vi "Format CSV.vi"(8 "error in (no error)":errorcluster, 9 "delimiter":string=",", 10 "CSV File Input":path, 11 "Original CSV Format":enum16{"Format A", "Format B"}(ring)) -> (0 "error out":errorcluster, 1 "Parcel Length":i32[](array[numeric]), 2 "All Terminal Data":T1(array[cluster]))   [LabVIEW 2017] (continued)
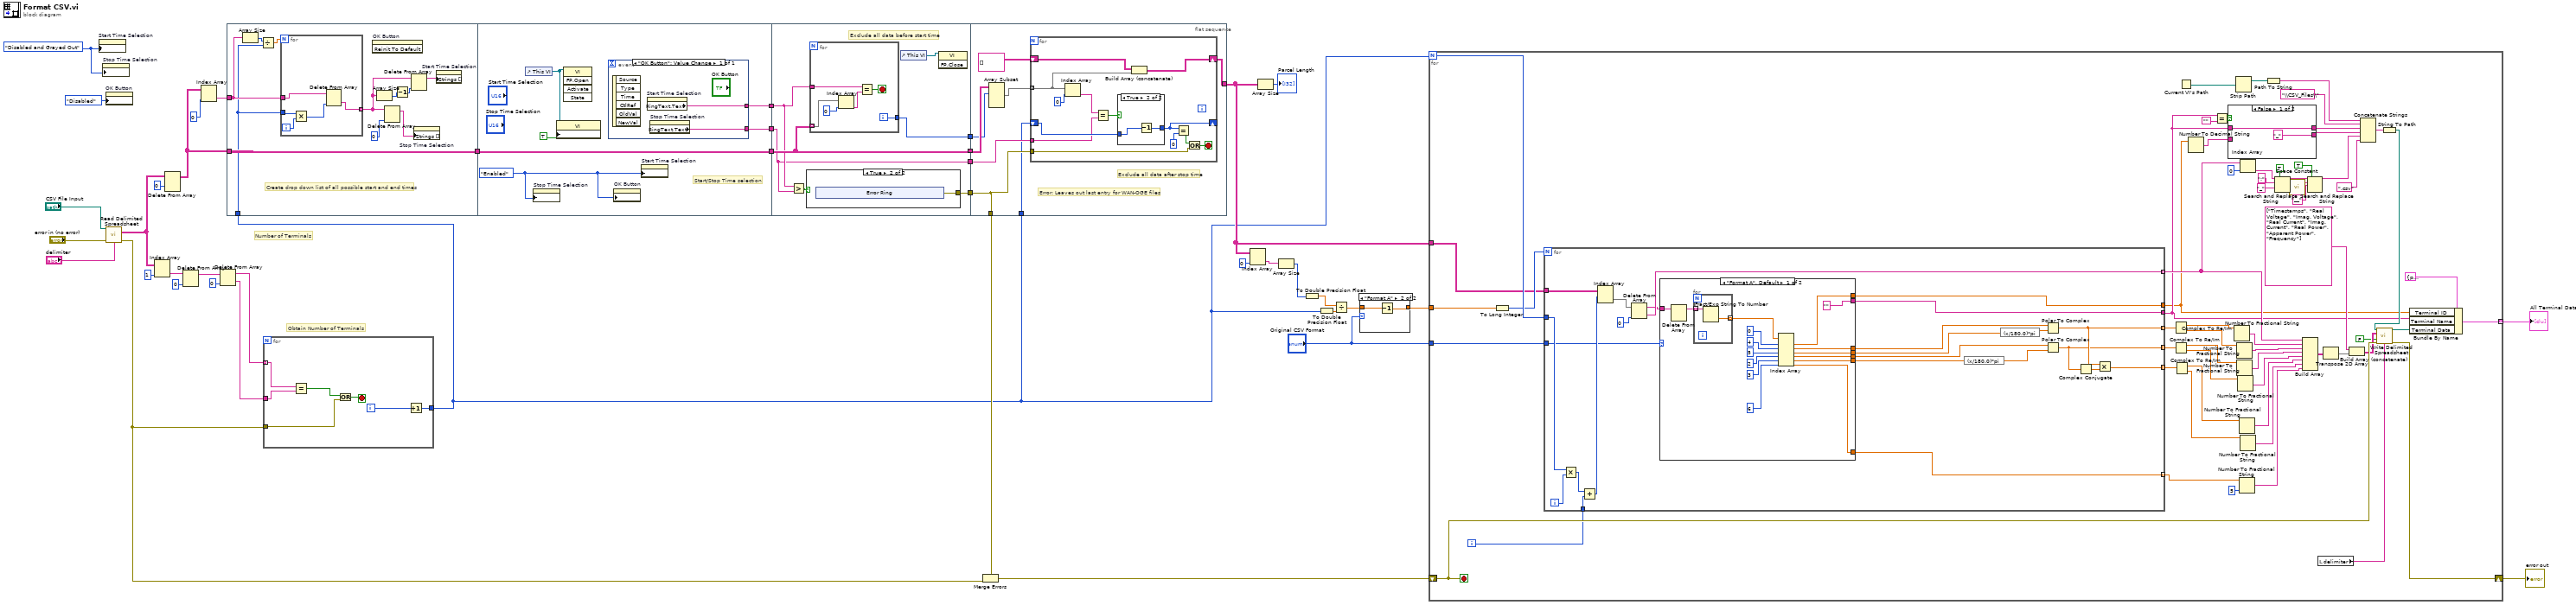
[diagram p0: block diagram]
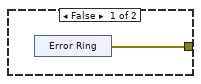
[diagram p3: hidden frame]
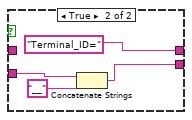
[diagram p5: hidden frame]
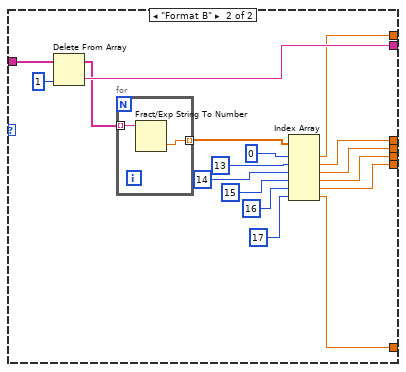
[diagram p6: hidden frame]
diagram:
  w3 = T2."Disabled and Grayed Out" ("Disabled")
  # "Obtain Number of Terminals"
  # "Number of Terminals"
  n1 = property on="Start Time Selection" class="Ring (strict)"("DisabledEnum"=w3) -> ()  [unwired: 2 in, 2 out]
  n2 = property on="Stop Time Selection" class="Ring (strict)"("DisabledEnum"=w3) -> ()  [unwired: 2 in, 2 out]
  n3 = property on="OK Button" class="Bool"("DisabledEnum"=T2."Disabled" ("Disabled")) -> ()  [unwired: 2 in, 2 out]
  n4 = call-poly <vilib>:"Read Delimited Spreadsheet.vi"("file path (dialog if empty)"="CSV File Input", "error in (no error)"="error in (no error)", "delimiter (\\t)"="delimiter") -> ("all rows"=w22:string[][], "error out"=w13:errorcluster)  [unwired: 7 in, 4 out]
  n5 = Index Array(array=w22, index (col)=1 ("disabled index (col)")) -> (element=w28:string[])  [unwired: 1 in]
  n6 = Delete From Array(array=w22, index (row)=0) -> (array with subset deleted=w20:string[][])  [unwired: 2 in, 1 out]
  n7 = Delete From Array(array=w28, index=0) -> (array with subset deleted=w27:string[])  [unwired: 1 in, 1 out]
  n8 = Index Array(array=w20, index (col)=0 ("disabled index (col)")) -> (element=w23:string[])  [unwired: 1 in]
  n9 = Delete From Array(array=w27, index=0) -> (deleted portion=w35:string, array with subset deleted=w36:string[])  [unwired: 1 in]
  n10 = flat-sequence {
    tunnel: [w52] -> w25
    tunnel: w20 -> [w52]
    tunnel: w23 -> [w51]
    tunnel: w4 -> [w46]
    tunnel: w25 -> [w63]
    tunnel: [w63] -> w19
    tunnel: [w60] -> w18
    tunnel: [w59] -> w17
    tunnel: w19 -> [w72]
    tunnel: w18 -> [w70]
    tunnel: w17 -> [w69]
    tunnel: [w69] -> w16
    tunnel: [w72] -> w15
    tunnel: [w71] -> w14
    tunnel: [w67] -> w11
    tunnel: [w94] -> w6
    tunnel: w16 -> [w91]
    tunnel: w15 -> [w92]
    tunnel: w14 -> [w90]
    tunnel: w4 -> [w87]
    tunnel: w11 -> [w88]
    tunnel: [w88] -> w10
    frame #0 {
      # "Create drop down list of all possible start and end times"
      n11 = Array Size(array=w51) -> (size(s)=w50:i32)
      n12 = Divide(x=w50, y=w46) -> (x/y=w49:dbl)
      n13 = for {
        N: w49 -> [_]
        tunnel: w51 -> [w55]
        tunnel: [w53] -> w45 mode=indexing
        tunnel: w46 -> [w56]
        i -> [w57]
        n14 = Multiply(x=w56, y=w57) -> (x*y=w54:i32)
        n15 = Delete From Array(array=w55, index=w54) -> (deleted portion=w53:string)  [unwired: 1 in, 1 out]
      }
      n16 = invoke on="OK Button" class="Bool" method="Reinit To Default"() -> ()  [unwired: 3 in, 3 out]
      n17 = Array Size(array=w45) -> (size(s)=w44:i32)
      n18 = Delete From Array(array=w45, index=0) -> (array with subset deleted=w47:string[])  [unwired: 1 in, 1 out]
      n19 = Decrement(x=w44) -> (x-1=w43:i32)
      n20 = Delete From Array(array=w45, index=w43) -> (array with subset deleted=w42:string[])  [unwired: 1 in, 1 out]
      n21 = property on="Stop Time Selection" class="Ring (strict)"("Strings []"=w47) -> ()  [unwired: 2 in, 2 out]
      n22 = property on="Start Time Selection" class="Ring (strict)"("Strings []"=w42) -> ()  [unwired: 2 in, 2 out]
    }
    frame #1 {
      w58 = T2."Enabled" ("Disabled")
      # "Start/Stop Time selection"
      n23 = control-ref of="This VI"() -> (w62:refnum<vi>)
      n24 = property on="Stop Time Selection" class="Ring (strict)"("DisabledEnum"=w58) -> ()  [unwired: 2 in, 2 out]
      n25 = property class="VI"(reference=w62, "Front Panel.IsFrontmost"=TRUE ("Front Panel Window:Is Frontmost")) -> ()  [unwired: 1 in, 2 out]
      n26 = invoke class="VI" method="FP.Open"(reference=w62) -> ()  [unwired: 4 in, 5 out]
      n27 = event shown="[0] \"OK Button\": Value Change" {
        selector: _ -> [_]
        dyn-events: _ -> [_]
        timeout: _ -> [_]
        tunnel: [w65] -> w60
        tunnel: [w64] -> w59
        event "OK Button": Value Change {
          n28 = event-data() -> ()  [unwired: 1 in, 6 out]
          n29 = property on="Start Time Selection" class="Ring (strict)"() -> ("RingText.Text"=w65:string)  [unwired: 2 in, 2 out]
          n30 = property on="Stop Time Selection" class="Ring (strict)"() -> ("RingText.Text"=w64:string)  [unwired: 2 in, 2 out]
        }
      }
      n31 = property on="OK Button" class="Bool"("DisabledEnum"=w58) -> ()  [unwired: 2 in, 2 out]
      n32 = property on="Start Time Selection" class="Ring (strict)"("DisabledEnum"=w58) -> ()  [unwired: 2 in, 2 out]
    }
    frame #2 {
      # "Exclude all data before start time"
      n33 = Greater?(x=w70, y=w69) -> (0:w68:bool)
      n34 = case shown="True" w68 {
        tunnel: [w73 w75] -> w67
        frame False {
          n35 = xnode "Error Ring"() -> ("error out"=w73:errorcluster)
        }
        frame True {
          n36 = xnode "Error Ring"() -> ("error out"=w75:errorcluster)
        }
      }
      n37 = for {
        tunnel: w72 -> [w85] mode=indexing
        tunnel: w70 -> [w83]
        tunnel: [w81] -> w71
        i -> [w81]
        stop <- w82 stop-if-true
        n38 = Index Array(array=w85, index=0) -> (element=w84:string)
        n39 = Equal?(x=w83, y=w84) -> (x = y?=w82:bool)
      }
      n40 = control-ref of="This VI"() -> (w66:refnum<vi>)
      n41 = invoke class="VI" method="FP.Close"(reference=w66) -> ()  [unwired: 2 in, 3 out]
    }
    frame #3 {
      # "Error: Leaves out last entry for WAN-OGE files"
      # "Exclude all data after stop time"
      n42 = Array Subset(array=w92, index (row)=w90) -> (w89:string[][])  [unwired: 3 in]
      n43 = for {
        shift-right: [w106] -> w94
        shift-left: string[][] [] ("all rows") -> [w107]
        tunnel: w91 -> [w96]
        tunnel: w89 -> [w103] mode=indexing
        tunnel: w88 -> [w97]
        shift-right: [w95] -> _
        shift-left: w87 -> [w100]
        stop <- w98 stop-if-true
        n44 = Index Array "Index Array"(array=w103, index=0) -> (element=w104:string)
        n45 = Equal?(x=w104, y=w96) -> (x = y?=w102:bool)
        n46 = case shown="True" w102 {
          tunnel: w100 -> [w108 w110]
          tunnel: [w108 w109] -> w95
          frame False {
          }
          frame True {
            n47 = Decrement(x=w110) -> (x-1=w109:i32)
          }
        }
        n48 = Build Array (concatenate)(w107, w103) -> (w106:string[][])
        n49 = Equal?(x=w95, y=0 ("index")) -> (x = y?=w99:bool)
        n50 = Or(x=w99, y=w97) -> (x .or. y?=w98:bool)
      }
    }
  }
  n51 = for {
    tunnel: w36 -> [w115] mode=indexing
    tunnel: w35 -> [w114]
    tunnel: [w116] -> w4
    tunnel: w13 -> [w113]
    i -> [w117]
    stop <- w111 stop-if-true
    n52 = Equal?(x=w115, y=w114) -> (x = y?=w112:bool)
    n53 = Or(x=w112, y=w113) -> (x .or. y?=w111:bool)
    n54 = Increment(x=w117) -> (x+1=w116:i32)
  }
  n55 = Merge Errors(w10, w13) -> (w12:errorcluster)
  n56 = Index Array(array=w6, index (col)=0 ("disabled index (col)")) -> (element=w32:string[])  [unwired: 1 in]
  n57 = Array Size(array=w6) -> (size(s)=→"Parcel Length":i32[])
  n58 = Array Size(array=w32) -> (size(s)=w31:i32)
  n59 = To Double Precision Float(number=w31) -> (double precision float=w29:dbl)
  n60 = To Double Precision Float(number=w4) -> (double precision float=w30:dbl)
  n61 = Divide(x=w29, y=w30) -> (x/y=w8:dbl)
  n62 = case shown="\"Format A\"" "Original CSV Format" {
    tunnel: w8 -> [w118 w120]
    tunnel: [w118 w119] -> w7
    frame "Format B" {
    }
    frame "Format A" {
      n63 = Decrement(x=w120) -> (x-1=w119:dbl)
    }
  }
  n64 = for {
    N: w4 -> [w178]
    shift-right: [w179] -> w41
    shift-left: w12 -> [w180]
    tunnel: w6 -> [w126]
    tunnel: "Original CSV Format" -> [w128]
    tunnel: w7 -> [w127]
    tunnel: [w173] -> w1 mode=indexing
    i -> [w177]
    stop <- w180 stop-if-true
    n65 = To Long Integer(number=w127) -> (32bit integer=w176:i32)
    n66 = for {
      N: w176 -> [_]
      tunnel: w126 -> [w190]
      tunnel: w128 -> [w204]
      tunnel: w178 -> [w210]
      tunnel: w177 -> [w208]
      tunnel: [w195] -> w171 mode=indexing
      tunnel: [w194] -> w170 mode=indexing
      tunnel: [w192] -> w169 mode=indexing
      tunnel: [w203] -> w132
      tunnel: [w188] -> w151 mode=indexing
      tunnel: [w202] -> w130
      tunnel: [w196] -> w162 mode=indexing
      i -> [w209]
      n67 = Multiply(x=w210, y=w209) -> (x*y=w207:i32)
      n68 = Add(x=w207, y=w208) -> (x+y=w206:i32)
      n69 = Index Array(array=w190, index (row)=w206) -> (element=w191:string[])  [unwired: 1 in]
      n70 = Delete From Array(array=w191, index=0 ("disabled index (col)")) -> (deleted portion=w188:string, array with subset deleted=w187:string[])  [unwired: 1 in]
      n71 = case shown="\"Format A\", Default" w204 {
        tunnel: w187 -> [w212 w244]
        tunnel: ["" ("String") w243] -> w203
        tunnel: [w219 w229] -> w202
        tunnel: [w217 w240] -> w201
        tunnel: [w216 w239] -> w200
        tunnel: [w215 w238] -> w199
        tunnel: [w214 w231] -> w197
        tunnel: [w213 w237] -> w196
        frame "Format A", Default {
          n72 = Delete From Array(array=w212) -> (array with subset deleted=w211:string[])  [unwired: 2 in, 1 out]
          n73 = for {
            tunnel: [w227] -> w225 mode=indexing
            tunnel: w211 -> [w228] mode=indexing
            n74 = Fract/Exp String To Number(string=w228) -> (number=w227:dbl)  [unwired: 3 in, 1 out]
          }
          n75 = Index Array(array=w225, index #1=0 ("index"), index #2=4 ("index"), index #3=5 ("index"), index #4=2 ("index"), index #5=3 ("index"), index #6=6 ("index")) -> (element #1=w219:dbl, element #2=w217:dbl, element #3=w216:dbl, element #4=w215:dbl, element #5=w214:dbl, element #6=w213:dbl)
        }
        frame "Format B" {
          n76 = Delete From Array(array=w244, index=1) -> (deleted portion=w243:string, array with subset deleted=w242:string[])  [unwired: 1 in]
          n77 = for {
            tunnel: [w246] -> w241 mode=indexing
            tunnel: w242 -> [w247] mode=indexing
            n78 = Fract/Exp String To Number(string=w247) -> (number=w246:dbl)  [unwired: 3 in, 1 out]
          }
          n79 = Index Array(array=w241, index #1=0 ("index"), index #2=13 ("index"), index #3=14 ("index"), index #4=15 ("index"), index #5=16 ("index"), index #6=17 ("index")) -> (element #1=w229:dbl, element #2=w240:dbl, element #3=w239:dbl, element #4=w238:dbl, element #5=w231:dbl, element #6=w237:dbl)
        }
      }
      n80 = expression code="(x/180.0)*pi" ("degrees to radians")(w197) -> (w198:dbl)
      n81 = expression code="(x/180.0)*pi" ("degrees to radians")(w200) -> (w205:dbl)
      n82 = Polar To Complex(1:w205, 2:w201) -> (0:w195:cdb)
      n83 = Polar To Complex(1:w198, 2:w199) -> (0:w194:cdb)
      n84 = Complex Conjugate(1:w194) -> (0:w193:cdb)
      n85 = Multiply(x=w195, y=w193) -> (x*y=w192:cdb)
    }
    n86 = Complex To Re/Im(x + iy=w171) -> (x=w163:dbl[], y=w164:dbl[])
    n87 = Complex To Re/Im(x + iy=w170) -> (x=w165:dbl[], y=w166:dbl[])
    n88 = Complex To Re/Im(x + iy=w169) -> (x=w167:dbl[], y=w168:dbl[])
    n89 = Current VI's Path() -> (path=w159:path)
    n90 = Number To Decimal String(number=w130) -> (decimal integer string=w129:string)  [unwired: 1 in]
    n91 = Equal?(x=w132, y="") -> (x = y?=w155:bool)
    n92 = case shown="False" w155 {
      tunnel: ["_" ("string") w184] -> w136
      tunnel: [w182 "Terminal_ID=" ("string")] -> w137
      tunnel: w132 -> [w182 _]
      tunnel: w129 -> [_ w186]
      frame False {
      }
      frame True {
        n93 = Concatenate Strings "Concatenate Strings"(w186, "__" ("string")) -> (w184:string)
      }
    }
    n94 = Number To Fractional String(number=w163) -> (F-format string=w150:string[])  [unwired: 3 in]
    n95 = Strip Path(path=w159) -> (stripped path=w160:path)  [unwired: 1 out]
    n96 = Number To Fractional String(number=w164) -> (F-format string=w149:string[])  [unwired: 3 in]
    n97 = Number To Fractional String(number=w165) -> (F-format string=w148:string[])  [unwired: 3 in]
    n98 = Number To Fractional String(number=w166) -> (F-format string=w147:string[])  [unwired: 3 in]
    n99 = Number To Fractional String(number=w167) -> (F-format string=w146:string[])  [unwired: 3 in]
    n100 = Number To Fractional String(number=w162, precision (6)=i16 5) -> (F-format string=w144:string[])  [unwired: 2 in]
    n101 = Index Array(array=w151, index=0) -> (element=w131:string)
    n102 = Number To Fractional String(number=w168) -> (F-format string=w145:string[])  [unwired: 3 in]
    n103 = Path To String(path=w160) -> (string=w153:string)
    n104 = Search and Replace String(replace all?=TRUE ("replace all? (F)"), input string=w131, search string=":", replace string="_" ("replace string (\"\")")) -> (result string=w122:string)  [unwired: 4 in, 3 out]
    n105 = call <vilib>:"Space Constant.vi"() -> ("String"=w121:string)
    n106 = Build Array(w151, w150, w149, w148, w147, w146, w145, w144) -> (w143:string[][])
    n107 = Search and Replace String(replace all?=TRUE ("replace all? (F)"), input string=w122, search string=w121, replace string="__" ("replace string (\"\")")) -> (result string=w123:string)  [unwired: 4 in, 3 out]
    n108 = local read "delimiter"() -> (w175:string)
    n109 = Transpose 2D Array(2D array=w143) -> (transposed array=w142:string[][])
    n110 = Build Array (concatenate)(string[] ["Timestamps", "Real Voltage", "Imag. Voltage", "Real Current", "Imag. Current", "Real Power", "Apparent Power", "Frequency"] ("Array"), w142) -> (w140:string[][])
    n111 = Concatenate Strings "Concatenate Strings"(w153, "\\CSV_Files\\" ("string"), w137, w136, w123, ".csv" ("string")) -> (w161:string)
    n112 = String To Path(string=w161) -> (path=w154:path)
    n113 = call-poly <vilib>:"Write Delimited Spreadsheet.vi"("file path (dialog if empty)"=w154, "2D data"=w140, "append to file? (new file:F)"=FALSE, "error in (no error)"=w180, "delimiter (\\t)"=w175) -> ("new file path (Not A Path if cancelled)"=w174:path, "error out"=w179:errorcluster)  [unwired: 9 in]
    n114 = Bundle By Name(cluster=T3 {"Terminal Data"=path "", "Terminal ID"=0.0, "Terminal Name"=""} ("Cluster"), "Terminal ID"=w130, "Terminal Name"=w132, "Terminal Data"=w174) -> (w173:T3)
  }
  "error out" <- w41
  "All Terminal Data" <- w1
